vi "Do.vi"(8 "error in (no error)":errorcluster, 10 "Actor in":refnum<class "Actor.lvclass">, 11 "PVUpdate-myDouble Msg":refnum<class "PVUpdate-myDouble Msg.lvclass">) -> (0 "error out":errorcluster, 2 "Actor out":refnum<class "Actor.lvclass">)   [LabVIEW 2013, in "PVClient-Example.lvlib" / "PVUpdate-myDouble Msg.lvclass"]
doc: "(<B>Filename</B>: Actor Framework.lvlib:Message.lvclass:Do.vi)\n\nDefines what a message does when it is received by an actor. Generally, a message instructs an actor to invoke one of its methods.\n\nBy default, this method does nothing. A child class must override it to define behavior. Create a child class by using the Actor Framework Message Maker dialog box."
uses:
  PVUpdate-myDouble Msg.lvclass
  <vilib>/ActorFramework/Actor/Actor.lvclass
  PVClient-Example/PVClient-Example.lvclass
  Core/Actors/CS++PVMonitor Messages/CS++PVUpdate Msg/CS++PVUpdate Msg.lvclass/CS++PVUpdate Msg.ctl
  Core/Classes/CS++ProcessVariables/ProcessVariable/PV.lvclass/PV.ctl
  Core/Classes/CS++ProcessVariables/ProcessVariable/PV.lvclass
  Core/Actors/CS++PVMonitor Messages/CS++PVUpdate Msg/CS++PVUpdate Msg.lvclass
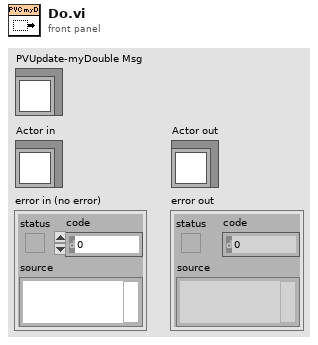
[diagram p1: front panel]
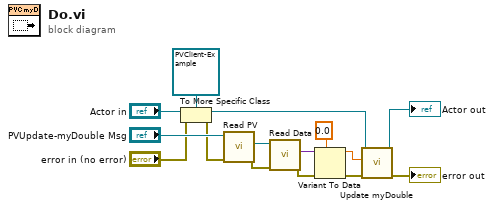
[diagram p0: block diagram]
diagram:
  n1 = To More Specific Class(target class=refnum<class "PVClient-Example.lvclass"> refnum ("PVClient-Example.lvlib:PVClient-Example.lvclass"), reference="Actor in", error in="error in (no error)") -> (specific class reference=w5:refnum<class "PVClient-Example.lvclass">, error out=w3:errorcluster)
  n2 = call "Read PV.vi"("error in (no error)"=w3, "CS++PVUpdate Msg in"="PVUpdate-myDouble Msg") -> ("error out"=w12:errorcluster, "PV"=w13:refnum<class "PV.lvclass">)  [unwired: 7 in, 1 out]
  n3 = call "Read Data.vi"("error in (no error)"=w12, "PV in"=w13) -> ("error out"=w11:errorcluster, "Data"=w9:variant)  [unwired: 7 in, 1 out]
  n4 = Variant To Data(error in=w11, type=0.0, Variant=w9) -> (data=w1:dbl, error out=w10:errorcluster)
  n5 = call "Update myDouble.vi"("error in (no error)"=w10, "myDouble"=w1, "PVClient-Example in"=w5) -> ("error out"=→"error out":errorcluster, "PVClient-Example out"=→"Actor out":refnum<class "PVClient-Example.lvclass">)  [unwired: 7 in]
